vi "PhotonCamera_SetDriverMode.vi"(9 "DriverMode":bool, 10 "BaseNTName":string="/photonvision", 11 "CameraName":string) -> (0 "error out":errorcluster)   [LabVIEW 2019, in "PhotonVisionLib.lvlib"]
doc: "Toggles driver mode.\n \nInputs:\n - cameraName -- The nickname of the camera (found in the PhotonVision UI).\n - DriverMode -- Whether to set driver mode.\nOutputs:\n - >none<"
uses:
  PhotonVisionLib.lvlib
  <vilib>/Rock Robotics/WPI/ThirdParty/JAS_Junk/TrajLib/VI/Util_GetTime_U32.vi
  <vilib>/Rock Robotics/WPI/ThirdParty/JAS_Junk/TrajLib/VI/Util_GetTime_U64.vi
  <vilib>/Rock Robotics/Network Tables/NT Read Boolean.vi
  <vilib>/Rock Robotics/Network Tables/NT Write Boolean.vi
  <vilib>/Rock Robotics/WPI/ThirdParty/JAS_Junk/TrajLib/Trajectory_Library.lvlib
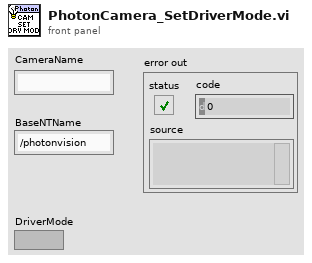
[diagram p1: front panel]
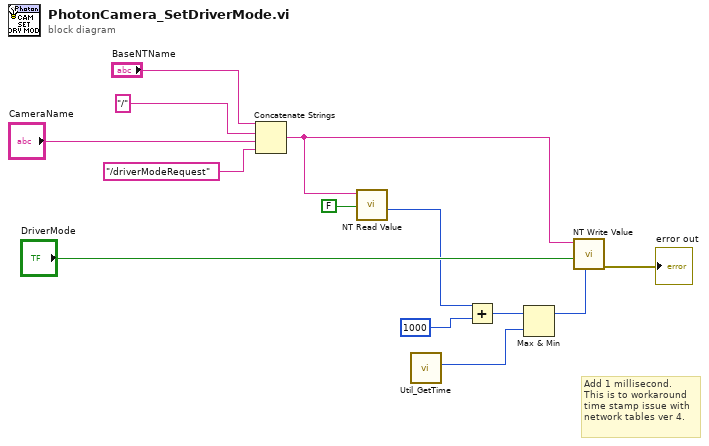
[diagram p0: block diagram]
diagram:
  # "Add 1 millisecond.\nThis is to workaround\ntime stamp issue with\nnetwork tables ver 4."
  n1 = Concatenate Strings("BaseNTName", "/", "CameraName", "/driverModeRequest") -> (w8:string)
  n2 = call-poly <vilib>:"NT Read Value.vi"("default value"=FALSE ("Default Value"), "name"=w8) -> ("timestamp"=w7:u64)  [unwired: 7 in, 2 out]
  n3 = call <vilib>:"Util_GetTime.vi"() -> ("FPGA_Time_MicroSeconds"=w3:u64)  [unwired: 9 in, 2 out]
  n4 = Add(x=w7, y=u64 1000) -> (x+y=w5:u64)
  n5 = Max & Min(x=w5, y=w3) -> (max(x,y)=w4:u64)  [unwired: 1 out]
  n6 = call-poly <vilib>:"NT Write Value.vi"("timestamp"=w4, "value"="DriverMode", "name"=w8) -> ("error out"=→"error out":errorcluster)  [unwired: 8 in]
